vi "Get_Disc_Flow_Rate.vi"(0 "Phase Average (mm)":dbl[][](array[numeric]), 5 "Radius (mm)":dbl[](array[numeric]), 11 "Jet Frequency":dbl) -> (2 "time":dbl[](array[numeric]), 3 "xd(t)":dbl[](array[numeric]), 4 "xd(t,r)":dbl[][](array[numeric]), 6 "Radius (m)":dbl[](array[numeric]), 8 "||xd||":dbl, 10 "||xd'||":dbl, 13 "beta":dbl[](array[numeric]), 14 "xd'(t)":dbl[](array[numeric]), 15 "||beta||":dbl)   [LabVIEW 2022 SP3]
uses:
  <vilib>/Analysis/2dsp.llb/Integral Method.ctl
  <vilib>/Analysis/1siggen.llb/Ramp Pattern by Samples.vi
  <vilib>/Analysis/baseanly.llb/Mean (DBL).vi
  <vilib>/Analysis/baseanly.llb/Scale 1D.vi
  <vilib>/Analysis/8numeric.llb/1D Numeric Integration.vi
  <vilib>/Analysis/NI_AALBase.lvlib
  <vilib>/gmath/NI_Gmath.lvlib
  <vilib>/Analysis/NI_AALPro.lvlib
panel:
  out "All Displacements":T1(graph)
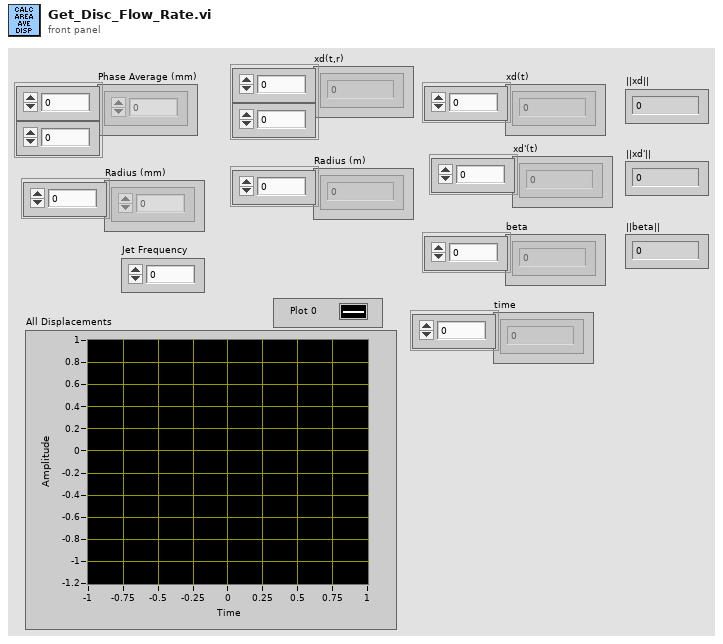
[diagram p1: front panel]
types:
  T1 = cluster{"Y=(X-offset)/scale":dbl[], "Y=(X-offset)/scale":dbl[]}[]
  T2 = typedef "NI_AALPro.lvlib/Integral Method.ctl" = i32
  T3 = cluster{"Y=(X-offset)/scale":dbl[], "Y=(X-offset)/scale":dbl[]}
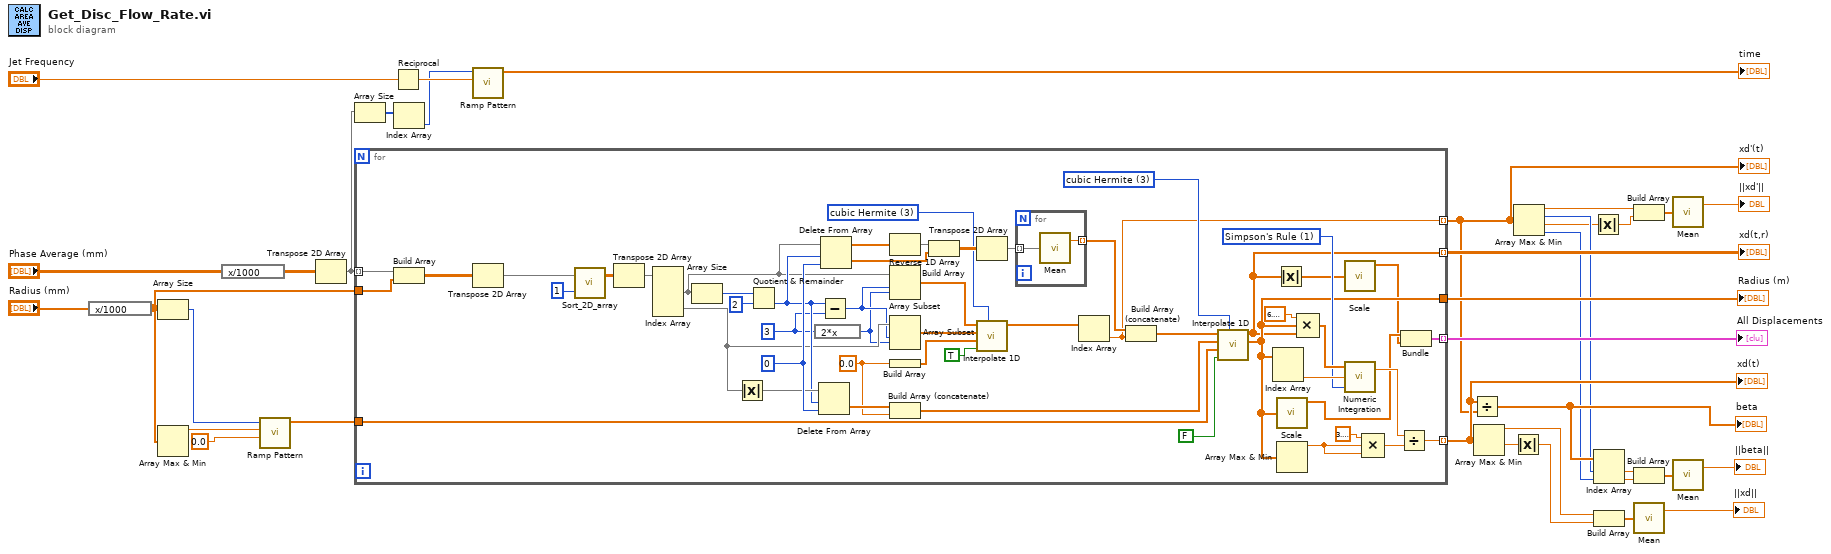
[diagram p0: block diagram]
diagram:
  n1 = expression code="x/1000"("Radius (mm)") -> (w27:dbl[])
  n2 = Array Size(array=w27) -> (size(s)=w28:i32)
  n3 = Array Max & Min(array=w27) -> (max value=w26:dbl)  [unwired: 3 out]
  n4 = expression code="x/1000"("Phase Average (mm)") -> (w30:dbl[][])
  n5 = call-poly <vilib>:"Ramp Pattern.vi"("start"=0.0, "end"=w26, "samples"=w28) -> ("Ramp Pattern"=w25:dbl[])  [unwired: 7 in, 1 out]
  n6 = Transpose 2D Array(2D array=w30) -> (transposed array=w33:dbl[][])
  n7 = Array Size(array=w33) -> (size(s)=w32:i32[])
  n8 = for {
    tunnel: w27 -> [w82]
    tunnel: w33 -> [w83] mode=indexing
    tunnel: w25 -> [w62]
    tunnel: [w51] -> w21 mode=indexing
    tunnel: [w50] -> w23
    tunnel: [w49] -> w22 mode=indexing
    tunnel: [w37] -> w1 mode=indexing
    tunnel: [w48] -> w19 mode=indexing
    w39 = 3 items=["nearest", "linear", "spline", "cubic Hermite", "Lagrange"] ("method")
    w56 = T2 1 items=["Trapezoidal Rule", "Simpson's Rule", "Simpson's 3/8 Rule", "Bode Rule"] ("integration method")
    w42 = 0.0
    w69 = 3 ("y")
    w75 = 0 ("index")
    w81 = 3 items=["nearest", "linear", "spline", "cubic Hermite", "Lagrange"] ("method")
    n9 = Build Array(w83, w82) -> (w84:dbl[][])
    n10 = Transpose 2D Array(2D array=w84) -> (transposed array=w86:dbl[][])
    n11 = call "Sort_2D_array.vi"("Column index to sort on"=1, "unsorted array"=w86) -> ("sorted array"=w87:dbl[][])  [unwired: 1 out]
    n12 = Transpose 2D Array(2D array=w87) -> (transposed array=w85:dbl[][])
    n13 = Index Array(array=w85) -> (element #1=w70:dbl[], element #2=w72:dbl[])  [unwired: 4 in]
    n14 = Array Size(array=w70) -> (size(s)=w79:i32)
    n15 = Absolute Value(x=w72) -> (abs(x)=w74:dbl[])
    n16 = Quotient & Remainder(x=w79, y=2) -> (floor(x/y)=w73:i32)  [unwired: 1 out]
    n17 = expression code="2*x"(w69) -> (w68:i32)
    n18 = Delete From Array(array=w74, length=w73, index=w75) -> (deleted portion=w63:dbl[])  [unwired: 1 out]
    n19 = Subtract(x=w73, y=w69) -> (x-y=w71:i32)
    n20 = Delete From Array(array=w70, length=w73, index=w75) -> (deleted portion=w66:dbl[], array with subset deleted=w67:dbl[])
    n21 = Reverse 1D Array(array=w67) -> (reversed array=w65:dbl[])
    n22 = Array Subset(array=w70, index=w71, length=w68) -> (w44:dbl[])
    n23 = Array Subset(array=w72, index=w71, length=w68) -> (w43:dbl[])
    n24 = Build Array(w42) -> (w41:dbl[])
    n25 = Build Array (concatenate)(w63, w42) -> (w60:dbl[])
    n26 = Build Array(w65, w66) -> (w77:dbl[][])
    n27 = Transpose 2D Array(2D array=w77) -> (transposed array=w76:dbl[][])
    n28 = call <vilib>:"Interpolate 1D.vi"("method"=w39, "X is monotonic"=TRUE, "xi"=w41, "X"=w43, "Y"=w44) -> ("yi"=w38:dbl[])  [unwired: 4 in, 2 out]
    n29 = for {
      tunnel: w76 -> [w90] mode=indexing
      tunnel: [w89] -> w64 mode=indexing
      n30 = call-poly <vilib>:"Mean.vi"("X"=w90) -> ("mean"=w89:dbl)  [unwired: 1 out]
    }
    n31 = Index Array(array=w38) -> (element=w37:dbl)  [unwired: 1 in]
    n32 = Build Array (concatenate)(w64, w37) -> (w61:dbl[])
    n33 = call <vilib>:"Interpolate 1D.vi"("method"=w81, "X is monotonic"=FALSE, "xi"=w62, "X"=w60, "Y"=w61) -> ("xi used"=w50:dbl[], "yi"=w49:dbl[])  [unwired: 4 in, 1 out]
    n34 = Index Array(array=w50) -> (element #2=w57:dbl)  [unwired: 2 in, 1 out]
    n35 = Absolute Value(x=w49) -> (abs(x)=w45:dbl[])
    n36 = call-poly <vilib>:"Scale.vi"("X"=w50) -> ("Y=(X-offset)/scale"=w47:dbl[])  [unwired: 3 out]
    n37 = Array Max & Min(array=w50) -> (max value=w55:dbl)  [unwired: 3 out]
    n38 = Compound Arithmetic op=MULTIPLY(6.283185307179586, w50, w49) -> (w58:dbl[])
    n39 = call-poly <vilib>:"Scale.vi"("X"=w45) -> ("Y=(X-offset)/scale"=w46:dbl[])  [unwired: 3 out]
    n40 = call-poly <vilib>:"Numeric Integration.vi"("integration method"=w56, "dt"=w57, "Input Array"=w58) -> ("result"=w53:dbl)  [unwired: 1 out]
    n41 = Compound Arithmetic op=MULTIPLY(3.141592653589793, w55, w55) -> (w52:dbl)
    n42 = Divide(x=w53, y=w52) -> (x/y=w51:dbl)
    n43 = Bundle("Y=(X-offset)/scale"=w47, "Y=(X-offset)/scale"=w46) -> (w48:T3)  [unwired: 1 in]
  }
  "xd(t)" <- w21
  "Radius (m)" <- w23
  "xd(t,r)" <- w22
  "xd'(t)" <- w1
  "All Displacements" <- w19
  n44 = Reciprocal(x="Jet Frequency") -> (1/x=w34:dbl)
  n45 = Index Array(array=w32) -> (element=w31:i32)  [unwired: 1 in]
  n46 = call-poly <vilib>:"Ramp Pattern.vi"("end"=w34, "samples"=w31) -> ("Ramp Pattern"=→"time":dbl[])  [unwired: 8 in, 1 out]
  n47 = Divide(x=w21, y=w1) -> (x/y=w18:dbl[])
  "beta" <- w18
  n48 = Array Max & Min(array=w21) -> (max value=w8:dbl, min value=w10:dbl)  [unwired: 2 out]
  n49 = Absolute Value(x=w10) -> (abs(x)=w9:dbl)
  n50 = Array Max & Min(array=w1) -> (max value=w3:dbl, max index (indices)=w17:i32, min value=w4:dbl, min index (indices)=w16:i32)
  n51 = Absolute Value(x=w4) -> (abs(x)=w6:dbl)
  n52 = Index Array(array=w18, index #1=w17, index #2=w16) -> (element #1=w14:dbl, element #2=w15:dbl)
  n53 = Build Array(w8, w9) -> (w11:dbl[])
  n54 = Build Array(w3, w6) -> (w5:dbl[])
  n55 = Build Array(w14, w15) -> (w13:dbl[])
  n56 = call-poly <vilib>:"Mean.vi"("X"=w11) -> ("mean"=→"||xd||":dbl)  [unwired: 1 out]
  n57 = call-poly <vilib>:"Mean.vi"("X"=w5) -> ("mean"=→"||xd'||":dbl)  [unwired: 1 out]
  n58 = call-poly <vilib>:"Mean.vi"("X"=w13) -> ("mean"=→"||beta||":dbl)  [unwired: 1 out]
